vi "getFrequencyViewer.vi"(8 "error in (no error)":errorcluster, 11 "frequencyCounterController.lvclass in":refnum<class "frequencyCounterController.lvclass">) -> (0 "error out":errorcluster, 2 "Hardware:FrequencyCounters:FrequencyViewer.lvclass":refnum<class "FrequencyViewer.lvclass">, 3 "frequencyCounterController.lvclass out":refnum<class "frequencyCounterController.lvclass">)   [LabVIEW 2011, in "Hardware.lvlib" / "frequencyCounters.lvlib" / "frequencyCounterController.lvclass"]
uses:
  frequencyCounterController.lvclass
  FrequencyViewer/FrequencyViewer.lvclass
  frequencyCounterController.lvclass/frequencyCounterController.ctl
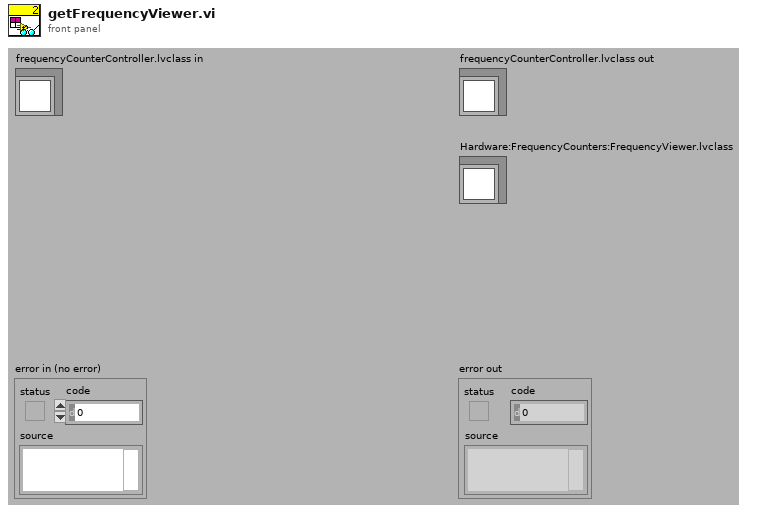
[diagram p1: front panel]
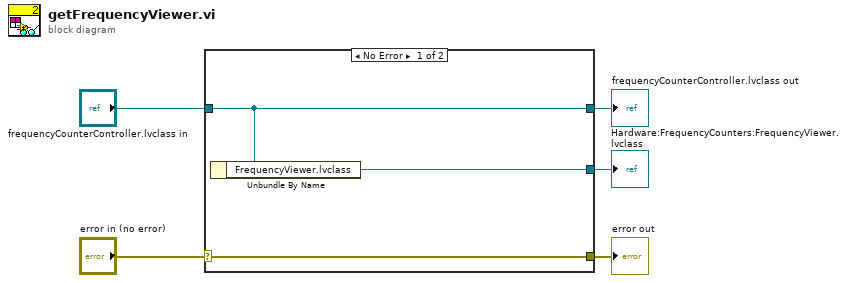
[diagram p0: block diagram]
diagram:
  n1 = case shown="No Error" "error in (no error)" {
    selector: "error in (no error)" -> [w8 w9]
    tunnel: [w8 w9] -> w4
    tunnel: [w7 w10] -> w2
    tunnel: "frequencyCounterController.lvclass in" -> [w7 w10]
    tunnel: [w6 _] -> w1
    frame No Error {
      n2 = Unbundle By Name(w7) -> ("FrequencyViewer.lvclass"=w6:refnum<class "FrequencyViewer.lvclass">)
    }
    frame Error {
    }
  }
  "error out" <- w4
  "frequencyCounterController.lvclass out" <- w2
  "Hardware:FrequencyCounters:FrequencyViewer.lvclass" <- w1
